vi "Get Variable Name.vi"(8 "error in (no error)":errorcluster, 11 "Variable URL":refnum<k21>) -> (0 "error out":errorcluster, 2 "Variable Name":string, 3 "dup Variable URL":refnum<k21>)   [LabVIEW 2024]
doc: "Gets the shared variable name from a shared variable URL."
uses:
  <resource>/objmgr/nvio.rc
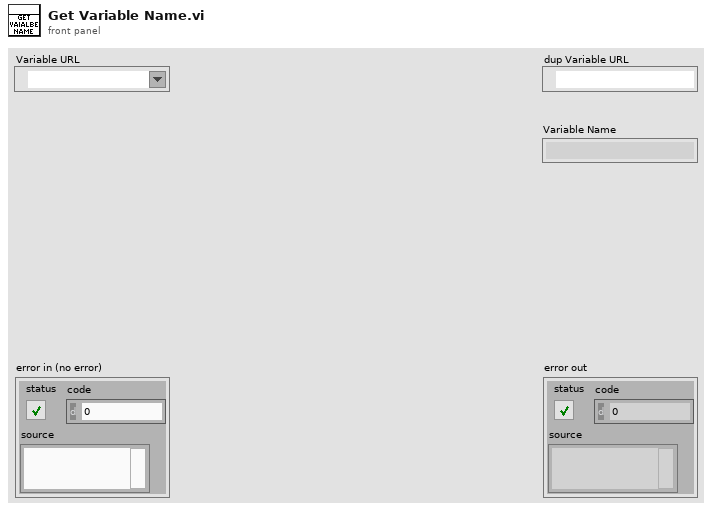
[diagram p1: front panel]
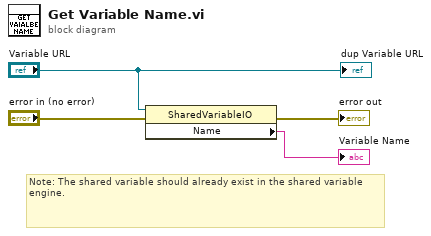
[diagram p0: block diagram]
diagram:
  # "Note: The shared variable should already exist in the shared variable engine."
  n1 = property class="SharedVariableIO"(reference="Variable URL", error in="error in (no error)") -> (error out=→"error out":errorcluster, "Name"=→"Variable Name":string)  [unwired: 1 out]
  "dup Variable URL" <- "Variable URL"
